vi "NI VeriStand - Report Final Error Status.vi"(8 "error in (no error)":errorcluster, 10 "Filter FIFO & Shutdown Errors (T)":bool=TRUE, 11 "Status Notifier":refnum<notifier>) -> (0 "error out":errorcluster)   [LabVIEW 2020, in "Custom Device Utility Library.lvlib"]
doc: "Reports a final error status from an asynchronous custom device to the VeriStand Engine. The VeriStand Engine checks the error status when the system shuts down."
uses:
  <vilib>/NI VeriStand/Custom Device Tools/Custom Device Utility Library/Custom Device Utility Library.lvlib
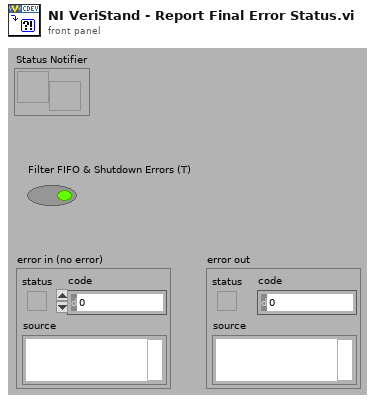
[diagram p1: front panel]
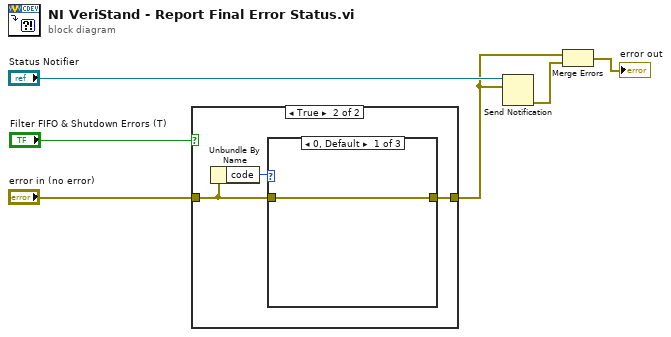
[diagram p0: block diagram]
diagram:
  n1 = case shown="True" "Filter FIFO & Shutdown Errors (T)" {
    tunnel: [w7 w9] -> w2
    tunnel: "error in (no error)" -> [w7 w8]
    frame False {
    }
    frame True {
      n2 = Unbundle By Name(w8) -> ("code"=w10:i32)
      n3 = case shown="0, Default" w10 {
        tunnel: [w11 _ _] -> w9
        tunnel: w8 -> [w11 _ _]
        frame 0, Default {
        }
        frame -2206 {
          # "This error is expected to be produced when the system is shutting down, because the system will kill the input and output FIFO references to signal the custom device to shut down."
        }
        frame -307557 {
          # "This error is expected to be produced when the system is shutting down."
        }
      }
    }
  }
  n4 = Send Notification(notification=w2, notifier="Status Notifier") -> (error out=w6:errorcluster)  [unwired: 1 in, 1 out]
  n5 = Merge Errors(w2, w6) -> (→"error out":errorcluster)
